vi "G-AI test harness.vi"(8 "error in":errorcluster) -> (0 "error out":errorcluster)   [LabVIEW 2020, in "G-AI tests.lvlib"]
uses:
  G-AI tests.lvlib
  src/G-AI Core/G-AI Core.lvlib
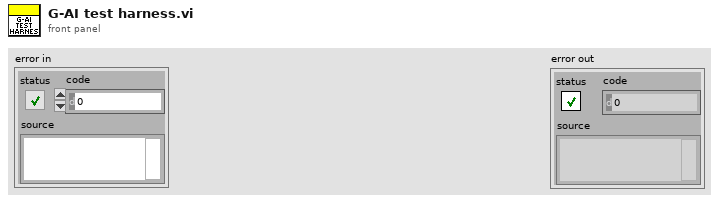
[diagram p1: front panel]
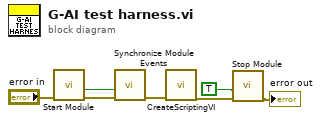
[diagram p0: block diagram]
diagram:
  n1 = call "Start Module.vi"("error in"="error in") -> ("error out"=w6:errorcluster, "Wait for Event Sync?"=w7:bool)  [unwired: 6 in, 3 out]
  n2 = call "Synchronize Module Events.vi"("error in"=w6, "Wait for Event Sync?"=w7) -> ("error out"=w5:errorcluster)  [unwired: 9 in]
  n3 = call "CreateScriptingVI.vi"("error in"=w5) -> ("error out"=w4:errorcluster)  [unwired: 10 in]
  n4 = call "Stop Module.vi"("error in"=w4, "Wait for Module to Stop? (F)"=TRUE) -> ("error out"=→"error out":errorcluster)  [unwired: 9 in]
